vi "数据标识输出.vi"(0 "运行模式":enum16{"按周期模式", "全常规模式"}(ring), 1 "时":i32) -> (14 "单位":string)   [LabVIEW 2016, in "流量计集成.lvlib"]
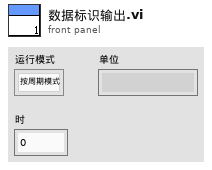
[diagram p1: front panel]
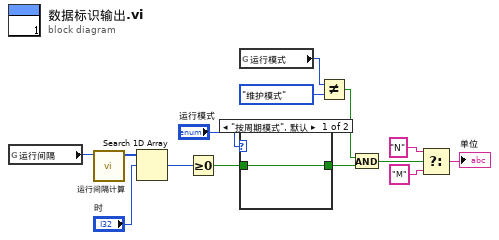
[diagram p0: block diagram]
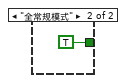
[diagram p2: hidden frame]
diagram:
  n1 = global read "流量计全局变量.vi" "运行间隔"() -> (w10:i16)
  n2 = call "运行间隔计算.vi"("运行周期"=w10) -> ("数组"=w13:i32[])  [unwired: 10 in]
  n3 = Search 1D Array(1D array=w13, element="时") -> (index of element=w12:i32)  [unwired: 1 in]
  n4 = Greater Or Equal To 0?(x=w12) -> (x >= 0?=w7:bool)
  n5 = global read "流量计全局变量.vi" "运行模式"() -> (w9:enum16{"维护模式", "常规模式", "应急模式", "质控模式", "性能测试"})
  n6 = case shown="\"按周期模式\", 默认" "运行模式" {
    tunnel: w7 -> [w15 _]
    tunnel: [w15 TRUE] -> w3
    frame "按周期模式", Default {
    }
    frame "全常规模式" {
    }
  }
  n7 = Not Equal?(x=w9, y=enum16{"维护模式", "常规模式", "应急模式", "质控模式", "性能测试"}."维护模式") -> (x != y?=w8:bool)
  n8 = And(x=w8, y=w3) -> (x .and. y?=w6:bool)
  n9 = Select(t="N" ("单位"), s=w6, f="M" ("单位")) -> (s? t:f=→"单位":string)
